vi "TB-Init Mic Queue.vi"(0 "state in":T4, 9 "Number":i32, 11 "error in (no error)":errorcluster, 13 "Pistonphone factor":dbl, 14 "Exposure parameters":T1={"Low cutoff (kHz)"=0.0, "High cutoff (kHz)"=0.0, "Duration (min)"=0.0, "dB SPL"=100.0, "Waveform"=enum."Noise", "WAVfile"=path "", "refWav"=path "", "use mic correction"=FALSE, "micCorrFile"=path "", "Pistonphone Level (dB SPL)"=0.0, "Sampling rate (Hz)"=0.0, "Buffer length (s)"=0.0, "Stream mic"=FALSE, "Fine adjust"={"Max"=0.0, "Min"=0.0}, "Mic gain"=0.0, "atten"=0.0, "resol (Hz)"=0.0, "navgs"=0, "Allow Slack"=FALSE, "max starts"=0, "Freq (kHz)"=8.0, "Tma (s)"=0.0, "Streamed"=[], "Drive"=""}) -> (4 "state out":T4, 6 "mic queue":T3, 15 "error out":errorcluster)   [LabVIEW 2020]
uses:
  Typedefs/TB-Runtime state.ctl
  <vilib>/sound2/lvsound2.llb/Sound File Refnum.ctl
  Typedefs/TB-Setup Log.ctl
  Typedefs/TB-Mic Queue.ctl
  Typedefs/TB-Parameters.ctl
  epl-vi-lib/Signal Synthesis VIs/Controls/Waveform XCtl/Waveform Enum.ctl
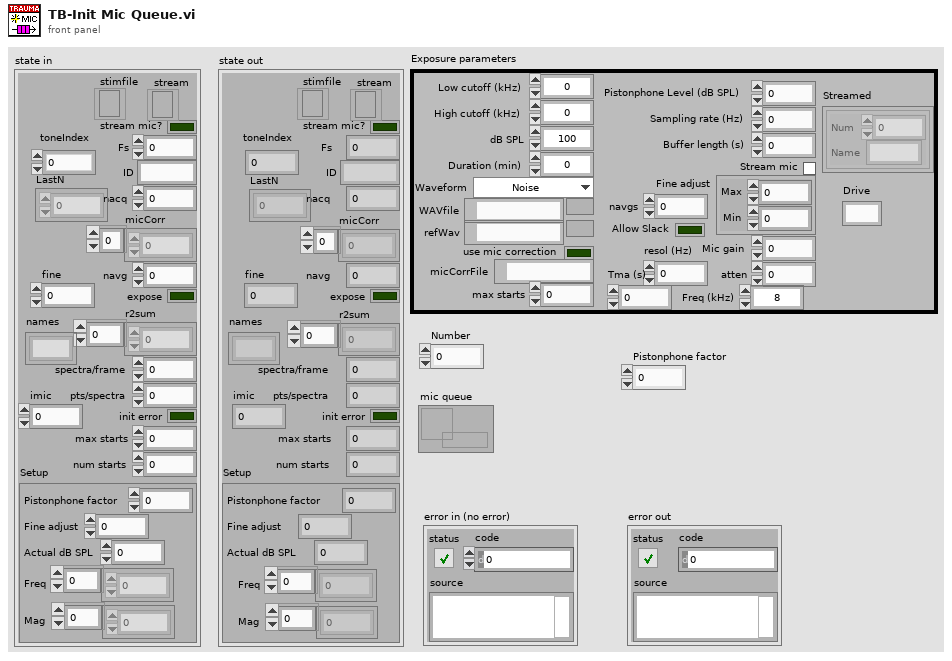
[diagram p1: front panel]
types:
  T1 = typedef "TB-Parameters.ctl" = cluster{"Low cutoff (kHz)":dbl, "High cutoff (kHz)":dbl, "Duration (min)":dbl, "dB SPL":dbl, "Waveform":T2, "WAVfile":path, "refWav":path, "use mic correction":bool, "micCorrFile":path, "Pistonphone Level (dB SPL)":dbl, "Sampling rate (Hz)":dbl, "Buffer length (s)":dbl, "Stream mic":bool, "Fine adjust":cluster{"Max":dbl, "Min":dbl}, "Mic gain":dbl, "atten":dbl, "resol (Hz)":dbl, "navgs":i32, "Allow Slack":bool, "max starts":i32, "Freq (kHz)":dbl, "Tma (s)":dbl, "Streamed":cluster{"Num":i32, "Name":string}[], "Drive":string}
  T2 = typedef "Waveform Enum.ctl" = enum16{"OFF", "Tone", "Noise", "Pulse Train", "File", "FM Sweep", "Chirp Train", "Complex Tone", "FM Tone", "Moving Ripple"}
  T3 = typedef "TB-Mic Queue.ctl" = refnum<queue>
  T4 = typedef "TB-Runtime state.ctl" = cluster{"stimfile":T5, "stream mic?":bool, "Fs":dbl, "ID":string, "micCorr":dbl[], "navg":i32, "r2sum":dbl[], "expose":bool, "spectra/frame":i32, "pts/spectra":i32, "nacq":i32, "init error":bool, "max starts":i32, "num starts":i32, "Setup":T6, "toneIndex":i32, "LastN":dbl[], "fine":dbl, "imic":i32, "stream":refnum<file>, "names":string[]}
  T5 = typedef "Sound File Refnum.ctl" = refnum<file>
  T6 = typedef "TB-Setup Log.ctl" = cluster{"Pistonphone factor":dbl, "Fine adjust":dbl, "Actual dB SPL":dbl, "Freq":dbl[], "Mag":dbl[]}
  T7 = enum16{"open", "replace", "create", "open or create", "replace or create", "replace or create with confirmation"}
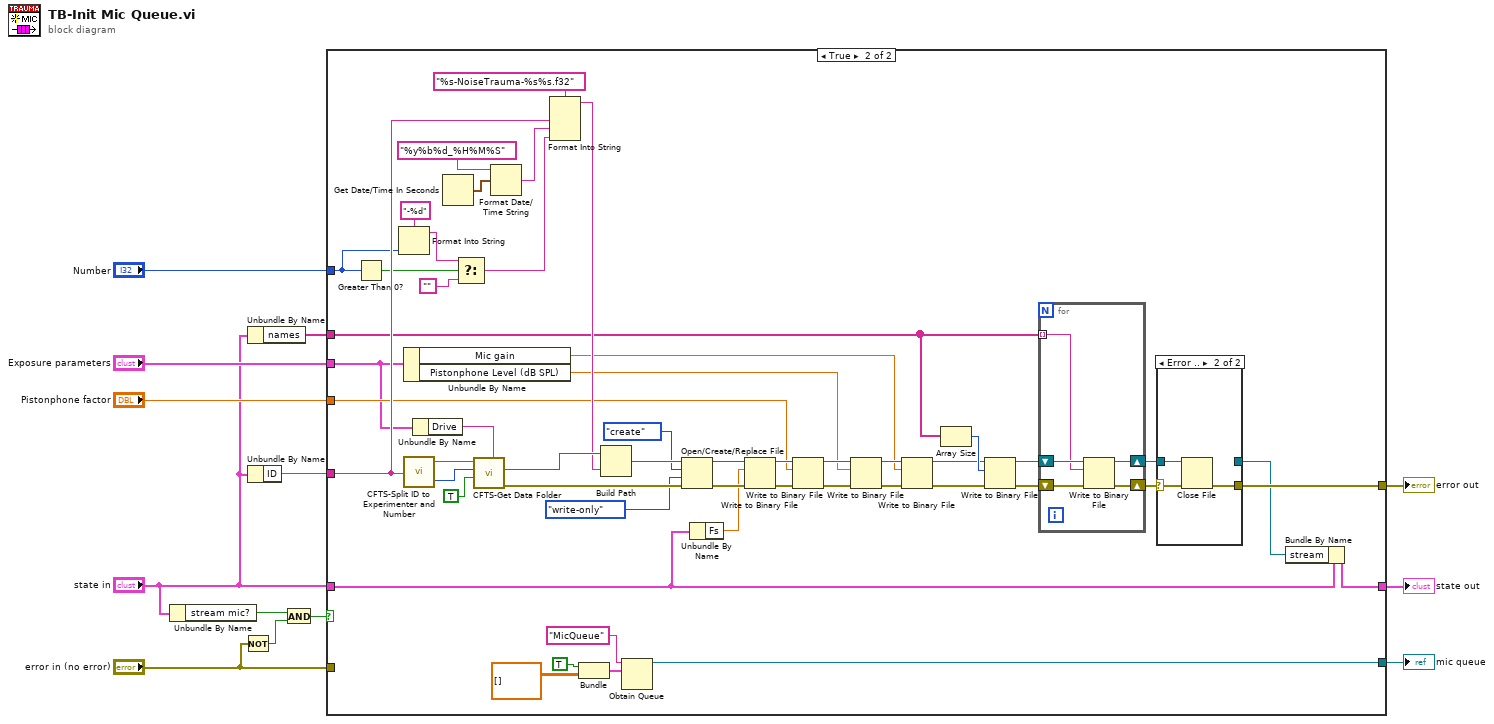
[diagram p0: block diagram]
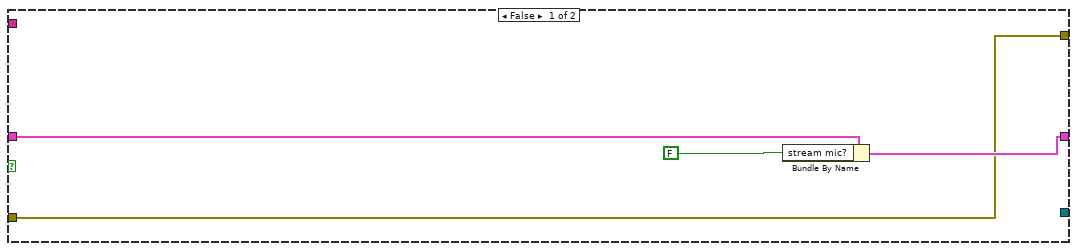
[diagram p2: hidden frame]
diagram:
  n1 = Unbundle By Name("state in") -> ("stream mic?"=w12:bool)
  n2 = Not(x="error in (no error)") -> (.not. x?=w13:bool)
  n3 = Unbundle By Name("state in") -> ("names"=w1:string[])
  n4 = Unbundle By Name("state in") -> ("ID"=w8:string)
  n5 = And(x=w12, y=w13) -> (x .and. y?=w10:bool)
  n6 = case shown="True" w10 {
    tunnel: [w16 w67] -> w7
    tunnel: "state in" -> [w17 w68]
    tunnel: w8 -> [_ w61]
    tunnel: [_ w52] -> w11
    tunnel: "error in (no error)" -> [w14 _]
    tunnel: "Number" -> [_ w46]
    tunnel: w1 -> [_ w35]
    tunnel: [w14 w32] -> w5
    tunnel: "Pistonphone factor" -> [_ w28]
    tunnel: "Exposure parameters" -> [_ w19]
    frame False {
      n7 = Bundle By Name(cluster=w17, "stream mic?"=FALSE ("micfile?")) -> (w16:T4)
    }
    frame True {
      n8 = Greater Than 0?(x=w46) -> (x > 0?=w50:bool)
      n9 = Format Into String(format string="-%d", w46) -> (resulting string=w47:string)  [unwired: 2 in, 1 out]
      n10 = Unbundle By Name(w19) -> ("Mic gain"=w21:dbl, "Pistonphone Level (dB SPL)"=w20:dbl)
      n11 = call "CFTS-Split ID to Experimenter and Number.vi"("ID"=w61) -> ("Experimenter"=w65:string, "Number"=w66:i32)
      n12 = Unbundle By Name(w19) -> ("Drive"=w18:string)
      n13 = Get Date/Time In Seconds() -> (seconds since 1Jan1904=w60:timestamp)
      n14 = Select(t=w47, s=w50, f="") -> (s? t:f=w48:string)
      n15 = call "CFTS-Get Data Folder.vi"("Drive"=w18, "create?"=TRUE, "Number"=w66, "Experimenter"=w65) -> ("error out"=w44:errorcluster, "Data folder"=w64:path)  [unwired: 6 in]
      n16 = Format Date/Time String(time format string (%c)="%y%b%d_%H%M%S", seconds (now)=w60) -> (date/time string=w58:string)  [unwired: 1 in]
      n17 = Format Into String(format string="%s-NoiseTrauma-%s%s.f32", w61, w58, w48) -> (resulting string=w62:string)  [unwired: 2 in, 1 out]
      n18 = Bundle(TRUE, dbl[][] []) -> (w55:cluster{bool, dbl[][]})  [unwired: 1 in]
      n19 = Build Path(base path=w64, name or relative path=w62) -> (appended path=w45:path)
      n20 = Obtain Queue(name (unnamed)="MicQueue", element data type=w55) -> (queue out=w52:refnum<queue>)  [unwired: 3 in, 2 out]
      n21 = Open/Create/Replace File(file path (use dialog)=w45, error in=w44, operation (0:open)=T7."create", access (0:read/write)=enum16{"read/write", "read-only", "write-only"}."write-only") -> (refnum out=w40:refnum<file>, error out=w41:errorcluster)  [unwired: 2 in, 1 out]
      n22 = Unbundle By Name(w68) -> ("Fs"=w39:dbl)
      n23 = Write to Binary File(file (use dialog)=w40, data=w39, error in=w41) -> (refnum out=w29:refnum<file>, error out=w30:errorcluster)  [unwired: 3 in, 1 out]
      n24 = Write to Binary File(file (use dialog)=w29, data=w28, error in=w30) -> (refnum out=w26:refnum<file>, error out=w27:errorcluster)  [unwired: 3 in, 1 out]
      n25 = Write to Binary File(file (use dialog)=w26, data=w20, error in=w27) -> (refnum out=w24:refnum<file>, error out=w25:errorcluster)  [unwired: 3 in, 1 out]
      n26 = Write to Binary File(file (use dialog)=w24, data=w21, error in=w25) -> (refnum out=w23:refnum<file>, error out=w22:errorcluster)  [unwired: 3 in, 1 out]
      n27 = Array Size(array=w35) -> (size(s)=w38:i32)
      n28 = Write to Binary File(file (use dialog)=w23, data=w38, error in=w22) -> (refnum out=w36:refnum<file>, error out=w37:errorcluster)  [unwired: 3 in, 1 out]
      n29 = for {
        shift-right: [w72] -> w34
        shift-left: w37 -> [w73]
        shift-right: [w70] -> w33
        shift-left: w36 -> [w71]
        tunnel: w35 -> [w69] mode=indexing
        n30 = Write to Binary File(file (use dialog)=w71, data=w69, error in=w73) -> (refnum out=w70:refnum<file>, error out=w72:errorcluster)  [unwired: 3 in, 1 out]
      }
      n31 = case shown="Error .." w34 {
        selector: w34 -> [w75 w78]
        tunnel: w33 -> [w74 w77]
        tunnel: [w75 w76] -> w32
        tunnel: [w74 _] -> w31
        frame No Error {
        }
        frame Error {
          n32 = Close File(refnum=w77, error in=w78) -> (error out=w76:errorcluster)  [unwired: 1 out]
        }
      }
      n33 = Bundle By Name(cluster=w68, "stream"=w31) -> (w67:T4)
    }
  }
  "error out" <- w5
  "state out" <- w7
  "mic queue" <- w11
